vi "Begin.vi"(8 "error in":errorcluster) -> (0 "error out":errorcluster)   [LabVIEW 2018]
doc: "Called before other user functions, this VI can be used to open I/O refnums, load in file data, and do general program initialization. Notice that the <B>error out</B> terminal is simply used for data flow. Wiring it to other structures or subVIs ensures that this VI runs first."
uses:
  <vilib>/Rock Robotics/WPI/DriverStation/WPI_DriverStationRobotMode2.ctl
  <vilib>/Rock Robotics/WPI/Joystick/WPI_JoystickDeviceEnum.ctl
  <vilib>/Rock Robotics/WPI/SafetyOutput/WPI_SafetyOutputConfigMenu.ctl
  <vilib>/Rock Robotics/SystemInterfaces/DIO/FPGA_DIOChannel.ctl
  <vilib>/Rock Robotics/WPI/Solenoid/WPI_SolenoidChannel.ctl
  Robot Global Data.vi
  <vilib>/Rock Robotics/Network Tables/NT Write String Array.vi
  <vilib>/Rock Robotics/WPI/RobotDrive/WPI_RobotDriveOpen4MotorWithExistingMotors.vi
  <vilib>/Rock Robotics/WPI/Switch/WPI_SwitchOpenLimit.vi
  <vilib>/Rock Robotics/WPI/Solenoid/WPI_SolenoidOpenDouble.vi
  <vilib>/Rock Robotics/WPI/Utilities/WPI_GetSetVariantRefNum.vi
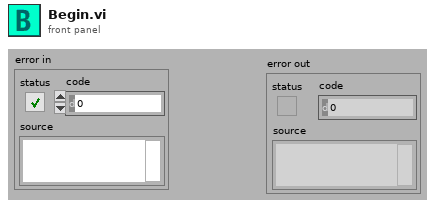
[diagram p1: front panel]
types:
  T1 = typedef "FPGA_DIOChannel.ctl" = enum8{"DIO 0", "DIO 1", "DIO 2", "DIO 3", "DIO 4", "DIO 5", "DIO 6", "DIO 7", "DIO 8", "DIO 9", "DIO MXP 0", "DIO MXP 1", "DIO MXP 2", "DIO MXP 3", "DIO MXP 4", "DIO MXP 5", "DIO MXP 6", "DIO MXP 7", "DIO MXP 8", "DIO MXP 9", "DIO MXP 10", "DIO MXP 11", "DIO MXP 12", "DIO MXP 13", "DIO MXP 14", "DIO MXP 15", "SPI Port CS1", "SPI Port CS2", "SPI Port CS3", "SPI Port MISO", "SPI Port MOSI", "Invalid"}
  T2 = typedef "WPI_SolenoidChannel.ctl" = enum8{"Solenoid 0", "Solenoid 1", "Solenoid 2", "Solenoid 3", "Solenoid 4", "Solenoid 5", "Solenoid 6", "Solenoid 7", "Invalid"}
  T3 = typedef "WPI_SafetyOutputConfigMenu.ctl" = enum16{"Enable", "Disable"}
  T4 = typedef "WPI_JoystickDeviceEnum.ctl" = enum16{"USB 0", "USB 1", "USB 2", "USB 3", "USB 4", "USB 5"}
  T5 = typedef "WPI_DriverStationRobotMode2.ctl" = enum16{"Autonomous Disabled", "Autonomous Enabled", "Teleop Disabled", "Teleop Enabled", "Disconnected", "Finish", "Test Disabled", "Test Enabled", "Emergency Stopped"}
  T6 = typedef "WPI_JoystickDevRef.ctl" = cluster{"Device":T4}
  T7 = typedef "WPI_MotorControlDeviceRef.ctl" = cluster{"DeviceStatus":errorcluster, "Type":T8, "PWM":cluster{"PWM Channel":T9, "DeadBand":T10}, "CAN":cluster{"Device Number":u8, "SetOutput VI Ref":variant, "GetOutput VI Ref":variant, "Enable VI Ref":variant, "Disable VI Ref":variant, "Data":variant}, "Invert":bool, "DIO PWM":cluster{"PWM \"Enable\" Channel":T9, "DIOChannel":T1, "PWM Rate":dbl}}
  T8 = typedef "WPI_MotorControlType.ctl" = enum16{"PWM", "CAN", "DIO PWM"}
  T9 = typedef "FPGA_DIOPWMChannel.ctl" = enum8{"PWM 0", "PWM 1", "PWM 2", "PWM 3", "PWM 4", "PWM 5", "PWM 6", "PWM 7", "PWM 8", "PWM 9", "PWM MXP 0", "PWM MXP 1", "PWM MXP 2", "PWM MXP 3", "PWM MXP 4", "PWM MXP 5", "PWM MXP 6", "PWM MXP 7", "PWM MXP 8", "PWM MXP 9", "Invalid"}
  T10 = typedef "WPI_PWMDeadband.ctl" = cluster{"Name":string, "maxPositivePwm":i32, "minPositivePwm":i32, "centerPwm":i32, "maxNegativePwm":i32, "minNegativePwm":i32, "angularRange":u16}
  T11 = typedef "WPI_RobotDriveDevRef.ctl" = cluster{"DevStatus":errorcluster, "Motors[]":T7[], "Square Inputs":bool, "Max Output":dbl}
  T12 = typedef "WPI_SwitchDevRef.ctl" = cluster{"DevStatus":errorcluster, "DIO Channel":T1, "CntIndex":T13, "Normally Closed":bool}
  T13 = typedef "FPGA_CounterCtrSystemIndex.ctl" = enum8{"Ctr 0", "Ctr 1", "Ctr 2", "Ctr 3", "Ctr 4", "Ctr 5", "Ctr 6", "Ctr 7", "Invalid"}
  T14 = typedef "WPI_CompressorDevRef.ctl" = cluster{"DevStatus":errorcluster, "Pneumatics Control Module":u8}
  T15 = typedef "WPI_SolenoidDevRef.ctl" = cluster{"DevStatus":errorcluster, "Pneumatics Control Module":u8, "Forward Solenoid Channel":T2, "Reverse Solenoid Channel":T2}
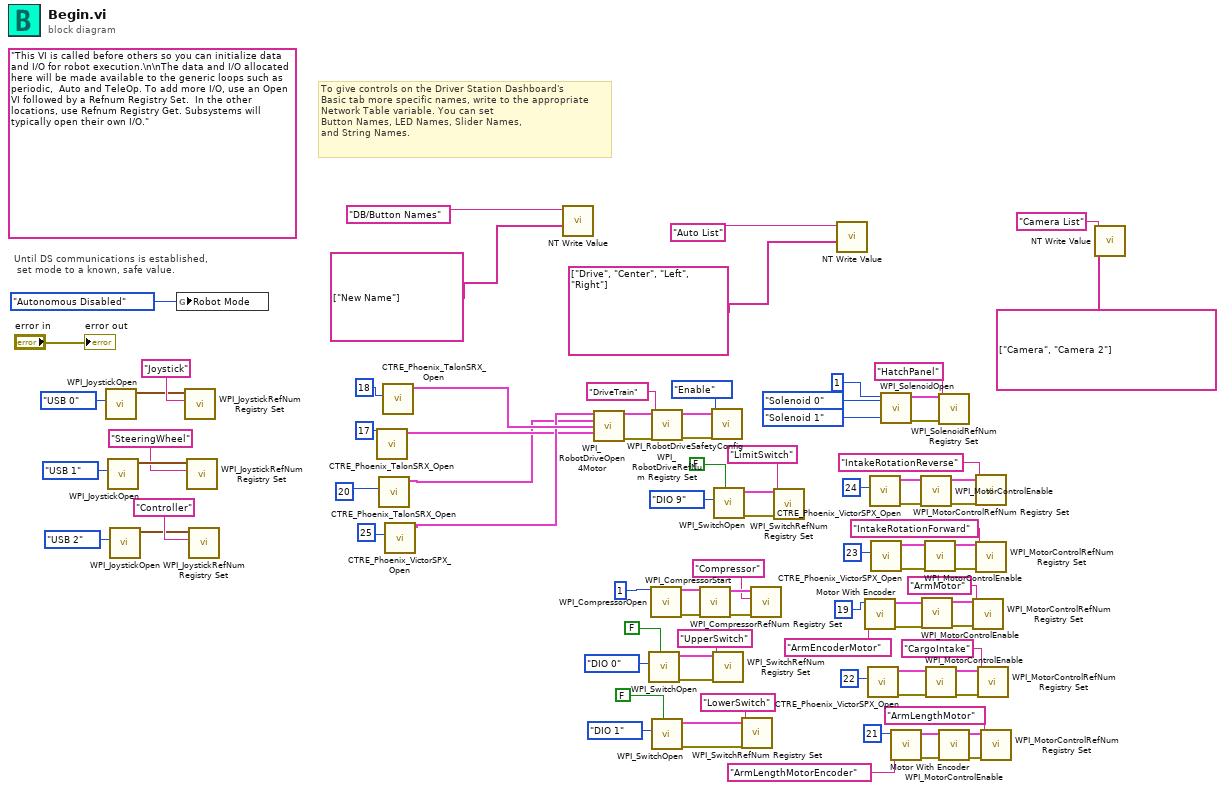
[diagram p0: block diagram]
diagram:
  (unwired) "This VI is called before others so you can initialize data and I/O for robot execution.\n\nThe data and I/O allocated here will be made available to the generic loops such as periodic,  Auto and TeleOp. To add more I/O, use an Open VI followed by a Refnum Registry Set.  In the other locations, use Refnum Registry Get. Subsystems will typically open their own I/O."
  # "To give controls on the Driver Station Dashboard's\nBasic tab more specific names, write to the appropriate\nNetwork Table variable. You can set\nButton Names, LED Names, Slider Names,\nand String Names."
  # "Until DS communications is established,\n set mode to a known, safe value."
  n1 = call <vilib>:"WPI_JoystickOpen.vi"("JoystickDevice"=WPI_JoystickDeviceEnum."USB 0") -> ("JoystickDevRef"=w88:T6)  [unwired: 10 in]
  n2 = call <vilib>:"WPI_JoystickOpen.vi"("JoystickDevice"=WPI_JoystickDeviceEnum."USB 1") -> ("JoystickDevRef"=w82:T6)  [unwired: 10 in]
  n3 = call <vilib>:"WPI_JoystickOpen.vi"("JoystickDevice"=WPI_JoystickDeviceEnum."USB 2") -> ("JoystickDevRef"=w79:T6)  [unwired: 10 in]
  n4 = global write "Robot Global Data.vi" "Robot Mode"(WPI_DriverStationRobotMode2."Autonomous Disabled" ("Robot Mode")) -> ()
  n5 = call <vilib>:"WPI_JoystickRefNum Registry Set.vi"("refnum name"="Joystick", "JoystickDevRef"=w88) -> ()  [unwired: 8 in, 2 out]
  n6 = call <vilib>:"WPI_JoystickRefNum Registry Set.vi"("refnum name"="SteeringWheel", "JoystickDevRef"=w82) -> ()  [unwired: 8 in, 2 out]
  n7 = call <vilib>:"WPI_JoystickRefNum Registry Set.vi"("refnum name"="Controller", "JoystickDevRef"=w79) -> ()  [unwired: 8 in, 2 out]
  n8 = call <vilib>:"CTRE_Phoenix_TalonSRX_Open.vi"("Device Number"=u8 17) -> ("CAN Talon SRX Ref"=w3:T7)  [unwired: 9 in, 1 out]
  n9 = call <vilib>:"CTRE_Phoenix_TalonSRX_Open.vi"("Device Number"=u8 20) -> ("CAN Talon SRX Ref"=w1:T7)  [unwired: 9 in, 1 out]
  n10 = call <vilib>:"CTRE_Phoenix_TalonSRX_Open.vi"("Device Number"=u8 18) -> ("CAN Talon SRX Ref"=w75:T7)  [unwired: 9 in, 1 out]
  n11 = call <vilib>:"CTRE_Phoenix_VictorSPX_Open.vi"("Device Number"=u8 25) -> ("CAN Talon SRX Ref"=w8:T7)  [unwired: 9 in, 1 out]
  n12 = call-poly <vilib>:"NT Write Value.vi"("String Array"=string[] ["New Name"], "Name"="DB/Button Names") -> ()  [unwired: 9 in, 1 out]
  n13 = call-poly <vilib>:"WPI_RobotDriveOpen4Motor.vi"("Rear Left Motor Dev Ref"=w8, "Rear Right Motor Dev Ref"=w1, "Front Left Motor Dev Ref"=w75, "Front Right Motor Dev Ref"=w3) -> ("RobotDriveDevRef"=w73:T11, "error out"=w74:errorcluster)  [unwired: 10 in]
  n14 = call-poly <vilib>:"WPI_SwitchOpen.vi"("Normally Closed"=FALSE, "DIO Channel"=FPGA_DIOChannel."DIO 0") -> ("error out"=w22:errorcluster, "SwitchDevRef"=w23:T12)  [unwired: 8 in]
  n15 = call <vilib>:"WPI_CompressorOpen.vi"("Pneumatics Control Module (0)"=u8 1) -> ("CompressorDevRef"=w32:T14, "error out"=w33:errorcluster)  [unwired: 13 in]
  n16 = call <vilib>:"WPI_RobotDriveRefNum Registry Set.vi"("error in (no error)"=w74, "refnum name"="DriveTrain", "RobotDriveDevRef"=w73) -> ("error out"=w71:errorcluster, "RobotDriveDevRef"=w70:T11)  [unwired: 7 in]
  n17 = call-poly <vilib>:"WPI_SwitchOpen.vi"("Normally Closed"=FALSE, "DIO Channel"=FPGA_DIOChannel."DIO 1") -> ("error out"=w21:errorcluster, "SwitchDevRef"=w20:T12)  [unwired: 8 in]
  n18 = call <vilib>:"WPI_CompressorStart.vi"("error in (no error)"=w33, "CompressorDevRef"=w32) -> ("error out"=w30:errorcluster, "CompressorDevRef"=w29:T14)  [unwired: 8 in]
  n19 = call <vilib>:"WPI_RobotDriveSafetyConfig.vi"("error in (no error)"=w71, "mode"=WPI_SafetyOutputConfigMenu."Enable", "RobotDriveDevRef"=w70) -> ()  [unwired: 7 in, 2 out]
  n20 = call <vilib>:"WPI_SwitchRefNum Registry Set.vi"("error in (no error)"=w22, "refnum name"="UpperSwitch", "SwitchDevRef"=w23) -> ()  [unwired: 7 in, 2 out]
  n21 = call-poly <vilib>:"WPI_SwitchOpen.vi"("Normally Closed"=FALSE, "DIO Channel"=FPGA_DIOChannel."DIO 9") -> ("error out"=w66:errorcluster, "SwitchDevRef"=w65:T12)  [unwired: 8 in]
  n22 = call <vilib>:"WPI_SwitchRefNum Registry Set.vi"("error in (no error)"=w21, "refnum name"="LowerSwitch", "SwitchDevRef"=w20) -> ()  [unwired: 7 in, 2 out]
  n23 = call <vilib>:"WPI_CompressorRefNum Registry Set.vi"("error in (no error)"=w30, "refnum name"="Compressor", "CompressorDevRef"=w29) -> ()  [unwired: 7 in, 2 out]
  n24 = call <vilib>:"WPI_SwitchRefNum Registry Set.vi"("error in (no error)"=w66, "refnum name"="LimitSwitch", "SwitchDevRef"=w65) -> ()  [unwired: 7 in, 2 out]
  n25 = call-poly <vilib>:"NT Write Value.vi"("String Array"=string[] ["Drive", "Center", "Left", "Right"], "Name"="Auto List") -> ()  [unwired: 9 in, 1 out]
  n26 = call "Motor With Encoder.vi"("refnum name"="ArmEncoderMotor", "Device Number"=u8 19) -> ("error out"=w50:errorcluster, "PhoenixMotorControlDevRef"=w49:T7)  [unwired: 8 in]
  n27 = call <vilib>:"CTRE_Phoenix_VictorSPX_Open.vi"("Device Number"=u8 22) -> ("error out"=w36:errorcluster, "CAN Talon SRX Ref"=w35:T7)  [unwired: 9 in]
  n28 = call <vilib>:"CTRE_Phoenix_VictorSPX_Open.vi"("Device Number"=u8 24) -> ("error out"=w54:errorcluster, "CAN Talon SRX Ref"=w53:T7)  [unwired: 9 in]
  n29 = call <vilib>:"CTRE_Phoenix_VictorSPX_Open.vi"("Device Number"=u8 23) -> ("error out"=w52:errorcluster, "CAN Talon SRX Ref"=w51:T7)  [unwired: 9 in]
  n30 = call-poly <vilib>:"WPI_SolenoidOpen.vi"("Reverse Solenoid Channel"=WPI_SolenoidChannel."Solenoid 1", "Forward Solenoid Channel"=WPI_SolenoidChannel."Solenoid 0", "Pneumatics Control Module (0)"=u8 1) -> ("error out"=w60:errorcluster, "SolenoidDevRef"=w59:T15)  [unwired: 7 in]
  n31 = call "Motor With Encoder.vi"("refnum name"="ArmLengthMotorEncoder", "Device Number"=u8 21) -> ("error out"=w12:errorcluster, "PhoenixMotorControlDevRef"=w11:T7)  [unwired: 8 in]
  n32 = call <vilib>:"WPI_MotorControlEnable.vi"("error in (no error)"=w54, "CAN MotorDevRef"=w53) -> ("error out"=w48:errorcluster, "CAN MotorDevRef"=w47:T7)  [unwired: 8 in]
  n33 = call <vilib>:"WPI_MotorControlEnable.vi"("error in (no error)"=w50, "CAN MotorDevRef"=w49) -> ("error out"=w39:errorcluster, "CAN MotorDevRef"=w38:T7)  [unwired: 8 in]
  n34 = call <vilib>:"WPI_MotorControlEnable.vi"("error in (no error)"=w52, "CAN MotorDevRef"=w51) -> ("error out"=w45:errorcluster, "CAN MotorDevRef"=w44:T7)  [unwired: 8 in]
  n35 = call <vilib>:"WPI_MotorControlEnable.vi"("error in (no error)"=w36, "CAN MotorDevRef"=w35) -> ("error out"=w42:errorcluster, "CAN MotorDevRef"=w41:T7)  [unwired: 8 in]
  n36 = call <vilib>:"WPI_SolenoidRefNum Registry Set.vi"("error in (no error)"=w60, "refnum name"="HatchPanel", "SolenoidDevRef"=w59) -> ()  [unwired: 7 in, 2 out]
  n37 = call <vilib>:"WPI_MotorControlEnable.vi"("error in (no error)"=w12, "CAN MotorDevRef"=w11) -> ("error out"=w16:errorcluster, "CAN MotorDevRef"=w15:T7)  [unwired: 8 in]
  n38 = call <vilib>:"WPI_MotorControlRefNum Registry Set.vi"("error in (no error)"=w39, "refnum name"="ArmMotor", "MotorControlDevRef"=w38) -> ()  [unwired: 7 in, 2 out]
  n39 = call <vilib>:"WPI_MotorControlRefNum Registry Set.vi"("error in (no error)"=w48, "refnum name"="IntakeRotationReverse", "MotorControlDevRef"=w47) -> ()  [unwired: 7 in, 2 out]
  n40 = call <vilib>:"WPI_MotorControlRefNum Registry Set.vi"("error in (no error)"=w45, "refnum name"="IntakeRotationForward", "MotorControlDevRef"=w44) -> ()  [unwired: 7 in, 2 out]
  n41 = call <vilib>:"WPI_MotorControlRefNum Registry Set.vi"("error in (no error)"=w42, "refnum name"="CargoIntake", "MotorControlDevRef"=w41) -> ()  [unwired: 7 in, 2 out]
  n42 = call <vilib>:"WPI_MotorControlRefNum Registry Set.vi"("error in (no error)"=w16, "refnum name"="ArmLengthMotor", "MotorControlDevRef"=w15) -> ()  [unwired: 7 in, 2 out]
  n43 = call-poly <vilib>:"NT Write Value.vi"("String Array"=string[] ["Camera", "Camera 2"], "Name"="Camera List") -> ()  [unwired: 9 in, 1 out]
  "error out" <- "error in"
